vi "Import OBJ.vi"(10 "Fill Colour":u32(colorbox), 11 "Object":path) -> (3 "Object":T1)   [LabVIEW 2022 SP3, in "3D.lvlib"]
uses:
  3D.lvlib
  Mesh.ctl
  Triangle 3D.ctl
  Vector 3D.ctl
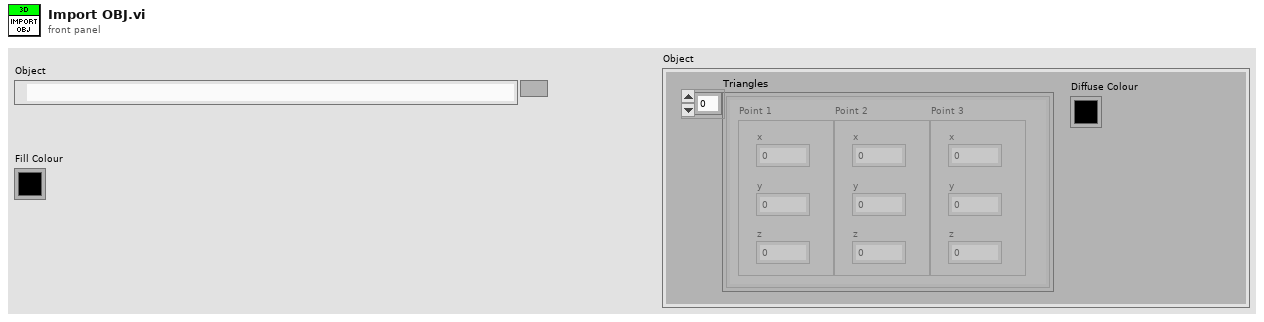
[diagram p1: front panel]
types:
  T1 = typedef "3D.lvlib/Mesh.ctl" = cluster{"Triangles":T2[], "Diffuse Colour":u32}
  T2 = typedef "3D.lvlib/Triangle 3D.ctl" = cluster{"Point 1":T3, "Point 2":T3, "Point 3":T3}
  T3 = typedef "3D.lvlib/Vector 3D.ctl" = cluster{"x":sgl, "y":sgl, "z":sgl}
  T4 = cluster{"default value 1":i32, "default value 1":i32, "default value 1":i32}
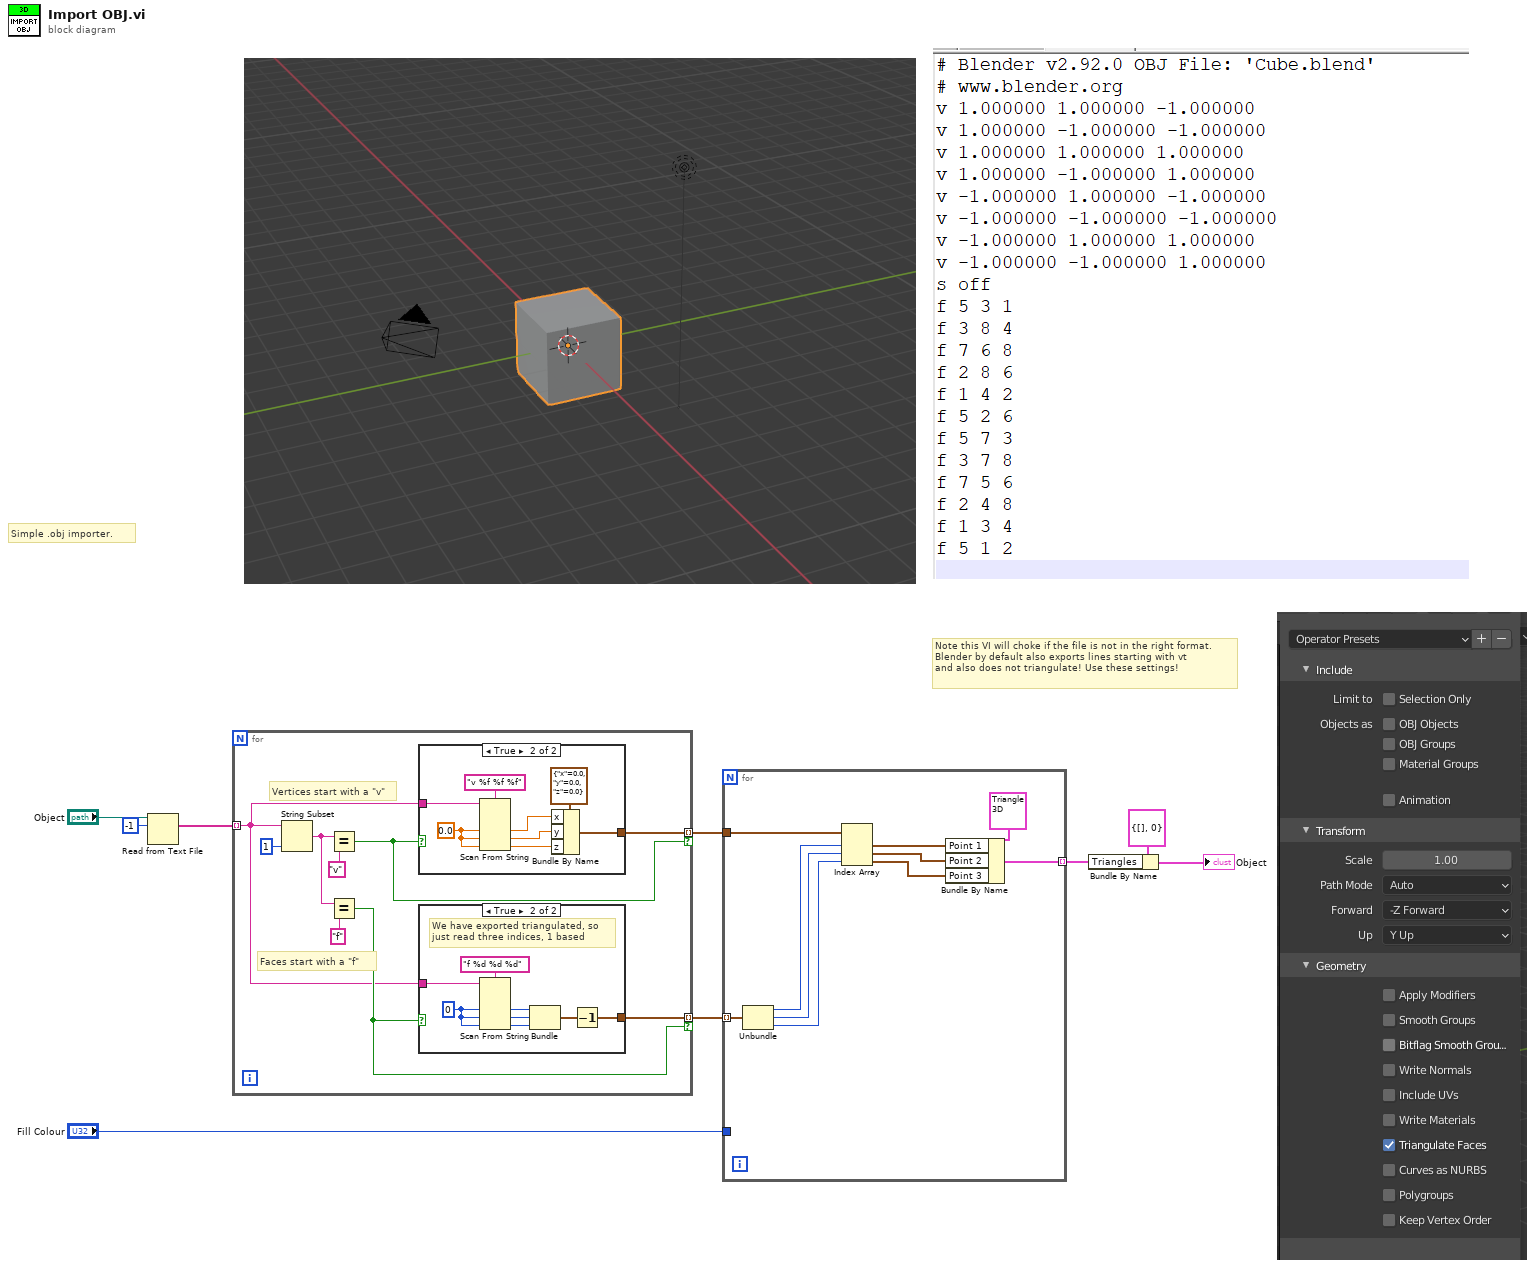
[diagram p0: block diagram]
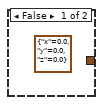
[diagram p2: hidden frame]
diagram:
  # "Note this VI will choke if the file is not in the right format. Blender by default also exports lines starting with vt\nand also does not triangulate! Use these settings!"
  # "Simple .obj importer."
  n1 = Read from Text File(file (use dialog)="Object", count=-1) -> (text=w7:string[])  [unwired: 2 in, 3 out]
  n2 = for {
    tunnel: w7 -> [w10] mode=indexing
    tunnel: [w15] -> w5 mode=indexing if=w14
    tunnel: [w12] -> w6 mode=indexing if=w11
    # "Faces start with a \"f\""
    # "Vertices start with a \"v\""
    n3 = String Subset(string=w10, length (rest)=1 ("length (rest)")) -> (substring=w13:string)  [unwired: 1 in]
    n4 = Equal?(x=w13, y="v") -> (x = y?=w14:bool)
    n5 = Equal?(x=w13, y="f") -> (x = y?=w11:bool)
    n6 = case shown="True" w14 {
      tunnel: w10 -> [_ w34]
      tunnel: [_ w27] -> w15
      frame False {
      }
      frame True {
        w32 = sgl 0.0 ("default value 1")
        n7 = Scan From String(format string="v %f %f %f", input string=w34, default 1=w32, default 2=w32, default 3=w32) -> (output 1=w30:sgl, output 2=w29:sgl, output 3=w28:sgl)  [unwired: 2 in, 3 out]
        n8 = Bundle By Name(cluster=T3 {"x"=0.0, "y"=0.0, "z"=0.0} ("Point 1"), "x"=w30, "y"=w29, "z"=w28) -> (w27:T3)
      }
    }
    n9 = case shown="True" w11 {
      tunnel: [_ w20] -> w12
      tunnel: w10 -> [_ w19]
      frame False {
        (unwired) T3 {"x"=0.0, "y"=0.0, "z"=0.0} ("Point 1")
      }
      frame True {
        w25 = 0 ("default value 1")
        # "We have exported triangulated, so just read three indices, 1 based"
        n10 = Scan From String(format string="f %d %d %d", input string=w19, default 1=w25, default 2=w25, default 3=w25) -> (output 1=w24:i32, output 2=w23:i32, output 3=w22:i32)  [unwired: 2 in, 3 out]
        n11 = Bundle("default value 1"=w24, "default value 1"=w23, "default value 1"=w22) -> (w21:T4)  [unwired: 1 in]
        n12 = Decrement(x=w21) -> (x-1=w20:T4)
      }
    }
  }
  n13 = for {
    tunnel: w6 -> [w44] mode=indexing
    tunnel: w5 -> [w42]
    tunnel: "Fill Colour" -> [_]
    tunnel: [w35] -> w1 mode=indexing
    n14 = Unbundle(w44) -> ("default value 1"=w41:i32, "default value 1"=w40:i32, "default value 1"=w39:i32)
    n15 = Index Array(array=w42, index #1=w41, index #2=w40, index #3=w39) -> (element #1=w38:T3, element #2=w37:T3, element #3=w36:T3)
    n16 = Bundle By Name(cluster=T2 {"Point 1"={"x"=0.0, "y"=0.0, "z"=0.0}, "Point 2"={"x"=0.0, "y"=0.0, "z"=0.0}, "Point 3"={"x"=0.0, "y"=0.0, "z"=0.0}} ("Triangle 2"), "Point 1"=w38, "Point 2"=w37, "Point 3"=w36) -> (w35:T2)
  }
  n17 = Bundle By Name(cluster=T1 {"Triangles"=[], "Diffuse Colour"=0} ("Object"), "Triangles"=w1) -> (→"Object":T1)
